vi "Test Method Hanging.vi"(8 "error in (no error)":errorcluster, 11 "Hanging Demo Case In":refnum<class "Hanging Dummy Case 2.lvclass">) -> (0 "error out":errorcluster, 3 "Hanging Demo Case Out":refnum<class "Hanging Dummy Case 2.lvclass">)   [LabVIEW 2020, in "Hanging Dummy Case.lvclass"]
uses:
  Hanging Dummy Case.lvclass
  Hanging Dummy Case 2/Hanging Dummy Case 2.lvclass
  C:/Users/anton/Documents/GitHub/LUnit/source/Framework/Test Case/LUnit Test Case.lvclass
  source/Framework/Test Case/LUnit Test Case.lvclass/LUnit Test Case.ctl
  source/Framework/Result Classes/Assertion Result/Assertion Result.lvclass/Assertion Result.ctl
  source/Framework/Result Classes/Test Case Result/Test Case Result.lvclass/Test Case Result.ctl
  source/Framework/Result Classes/Method Result/Method Result.lvclass/Method Result.ctl
  source/Framework/Test Case/Private/SubVIs/Add test result.vi
  source/Framework/Result Classes/Assertion Result/Community/Write Passed.vi
  source/Framework/Result Classes/Assertion Result/Community/Write Message.vi
  source/Framework/Result Classes/Assertion Result/Community/Write Description.vi
  source/Framework/Test Case/Private/SubVIs/Set Assertion Type.vi
  source/Framework/Result Classes/Test Case Result/Community/Record Assertion Result.vi
  source/Framework/Result Classes/Assertion Result/Community/Write Assertion Type.vi
  source/Framework/Result Classes/Method Result/Community/Accessors/Aggregate Assertion Results.vi
  source/Framework/Result Classes/Assertion Result/Public/Read Status.vi
  source/Framework/Result Classes/Assertion Result/Public/Read Message.vi
  source/Framework/Result Classes/Assertion Result/Public/Read Description.vi
  source/Framework/Result Classes/Method Result/Private/SubVIs/Merge Status.vi
  source/Framework/Result Classes/Method Result/Private/SubVIs/Concatenate result strings.vi
  source/Framework/Result Classes/Assertion Result/Assertion Result.lvclass
  source/Framework/Test Case/LUnit Test Case.lvclass
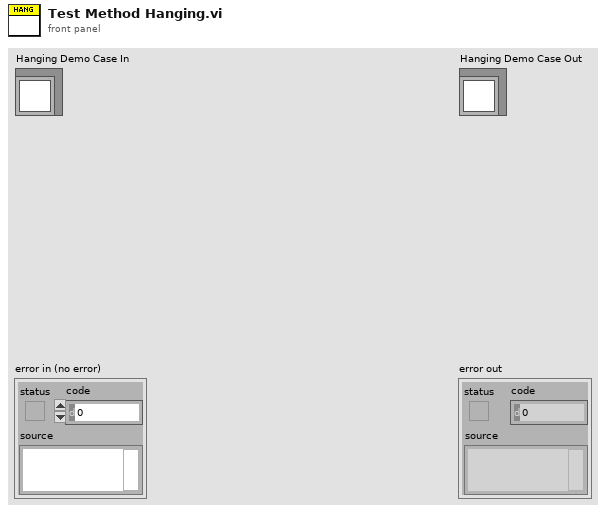
[diagram p1: front panel]
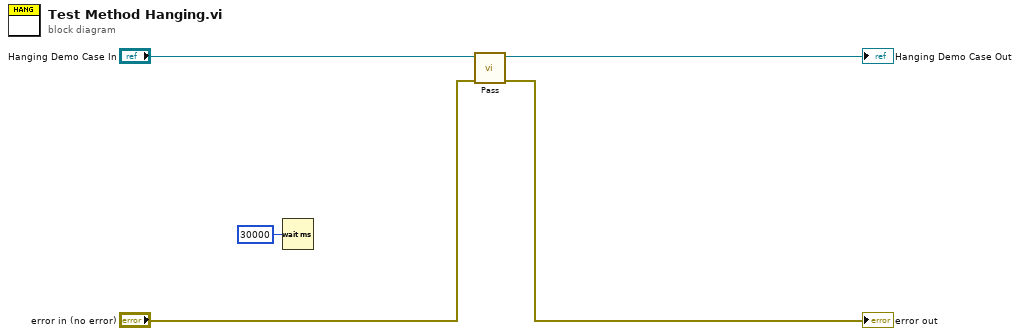
[diagram p0: block diagram]
diagram:
  n1 = Wait (ms)(milliseconds to wait=u32 30000) -> ()  [unwired: 1 out]
  n2 = call "Pass.vi"("error in (no error)"="error in (no error)", "LUnit Test Case In"="Hanging Demo Case In") -> ("error out"=→"error out":errorcluster, "LUnit Test Case Out"=→"Hanging Demo Case Out":refnum<class "Hanging Dummy Case 2.lvclass">)  [unwired: 8 in]
